vi "Set Buffer Size.vi"(0 "VISA resource name":refnum<visa-resource-name>, 5 "Buffer Name (defbuffer1)":string="defbuffer1", 7 "Buffer Size":u16, 11 "error in (no error)":errorcluster) -> (4 "VISA resource name out":refnum<visa-resource-name>, 15 "error out":errorcluster)   [LabVIEW 2020, in "Keithley 2450.lvlib"]
doc: "This sets the number of readings a buffer can store or sets a new number of readings that an already existing buffer can store."
uses:
  <instrlib>/Keithley 2450/Keithley 2450.lvlib
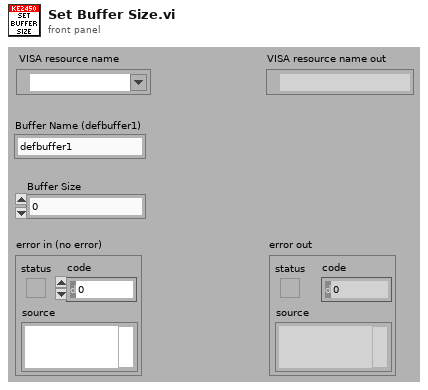
[diagram p1: front panel]
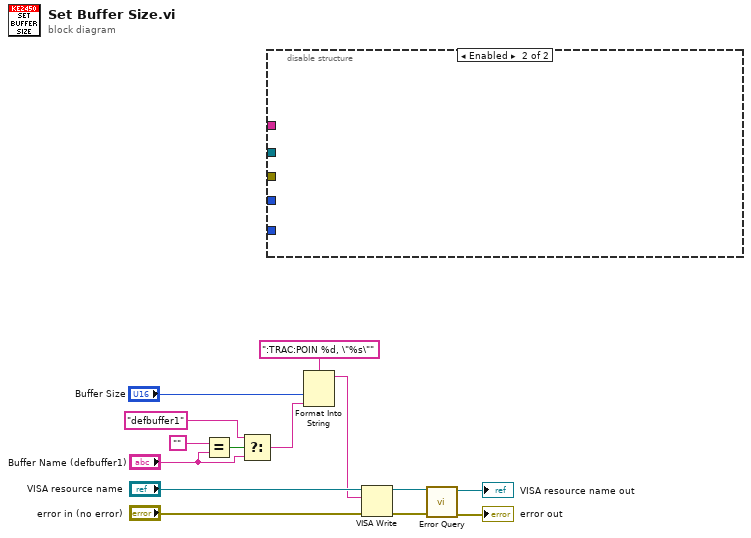
[diagram p0: block diagram]
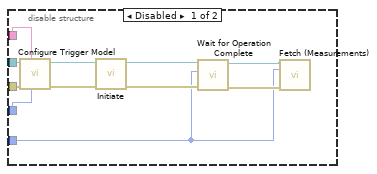
[diagram p2: hidden frame]
diagram:
  n1 = Equal?(x="", y="Buffer Name (defbuffer1)") -> (x = y?=w11:bool)
  n2 = Select(t="defbuffer1", s=w11, f="Buffer Name (defbuffer1)") -> (s? t:f=w2:string)
  n3 = disable-structure shown="Enabled" {
    disable-tunnel: _ -> [w21 _]
    disable-tunnel: _ -> [w20 _]
    disable-tunnel: _ -> [w19 _]
    disable-tunnel: _ -> [w18 _]
    disable-tunnel: _ -> [w15 _]
    frame Disabled {
      n4 = call <instrlib>:"Configure Trigger Model.vi"("Trigger Count (1)"=w20, "Buffer Name (defbuffer1)"=w15, "error in (no error)"=w18, "VISA resource name"=w19) -> ("error out"=w16:errorcluster, "VISA resource name out"=w17:refnum<visa-resource-name>)  [unwired: 6 in]
      n5 = call <instrlib>:"Initiate.vi"("error in (no error)"=w16, "VISA resource name"=w17) -> ("error out"=w24:errorcluster, "VISA resource name out"=w25:refnum<visa-resource-name>)  [unwired: 8 out]
      n6 = call <instrlib>:"Wait for Operation Complete.vi"("error in (no error)"=w24, "Timeout (10000 ms)"=w21, "VISA resource name"=w25) -> ("error out"=w23:errorcluster, "VISA resource name out"=w22:refnum<visa-resource-name>)  [unwired: 7 out]
      n7 = call <instrlib>:"Fetch (Measurements).vi"("VISA resource name"=w22, "Timeout (10000 ms)"=w21, "error in (no error)"=w23) -> ()  [unwired: 2 in, 11 out]
    }
    frame Enabled {
    }
  }
  n8 = Format Into String(format string=":TRAC:POIN %d, \"%s\"" ("Fetch Measurement"), "Buffer Size", w2) -> (resulting string=w3:string)  [unwired: 2 in, 1 out]
  n9 = VISA Write(VISA resource name="VISA resource name", write buffer=w3, error in (no error)="error in (no error)") -> (VISA resource name out=w6:refnum<visa-resource-name>, error out=w5:errorcluster)  [unwired: 1 out]
  n10 = call <instrlib>:"Error Query.vi"("error in (no error)"=w5, "VISA resource name"=w6) -> ("error out"=→"error out":errorcluster, "VISA resource name out"=→"VISA resource name out":refnum<visa-resource-name>)  [unwired: 8 out]
